vi "close_vi.vi"(1 "Process Stop Button":bool, 2 "reference":refnum<vi>) -> (0 "error out":errorcluster)   [LabVIEW 2015]
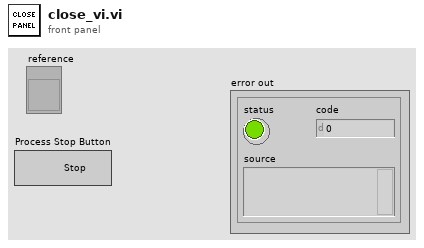
[diagram p1: front panel]
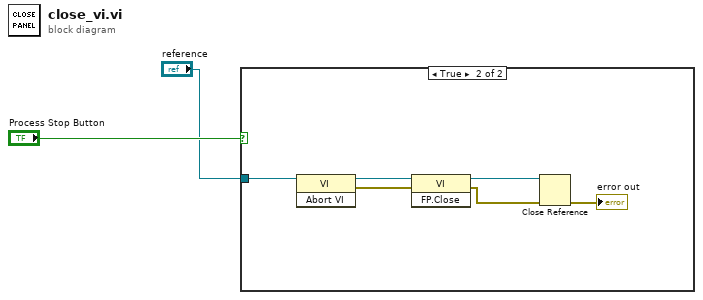
[diagram p0: block diagram]
diagram:
  n1 = case shown="True" "Process Stop Button" {
    tunnel: "reference" -> [_ w4]
    frame False {
    }
    frame True {
      n2 = invoke class="VI" method="Abort VI"(reference=w4) -> (reference out=w5:refnum<vi>, error out=w3:errorcluster)  [unwired: 2 in, 1 out]
      n3 = invoke class="VI" method="FP.Close"(reference=w5, error in=w3) -> (reference out=w8:refnum<vi>, error out=w7:errorcluster)  [unwired: 1 in, 1 out]
      n4 = Close Reference(reference=w8, error in (no error)=w7) -> (error out=→"error out":errorcluster)
    }
  }
